vi "Append Text Table to Report.vi"(0 "report in":refnum<class "NI_Excel.lvclass">, 1 "column width (1)":dbl=1.0 format="%.2f", 2 "measurement system":u16(ring)=2 caption="measurement system for column width (Default)" items=["US", "Metric", "Default"], 3 "MS Office parameters":T2, 5 "column headers":string[](array[string]), 7 "row headers":string[](array[string]), 9 "text data":string[][](array[string]), 11 "error in (no error)":errorcluster, 13 "separate page?":bool, 14 "show grid lines":bool=TRUE) -> (4 "report out":refnum<class "NI_Excel.lvclass">, 8 "range (wd) - start (xl)":T1, 10 "end (xl)":cluster{"row (xl) ":i32, "col (xl) ":i32}, 15 "error out":errorcluster)   [LabVIEW 2023, in "NI_Excel.lvclass"]
doc: "Appends a 2D array to a report as a table with the given column width. You can use this polymorphic VI to append an array of strings or numbers. The data type you wire to the <B>text data</B> input determines the polymorphic instance to use."
uses:
  NI_Excel.lvclass
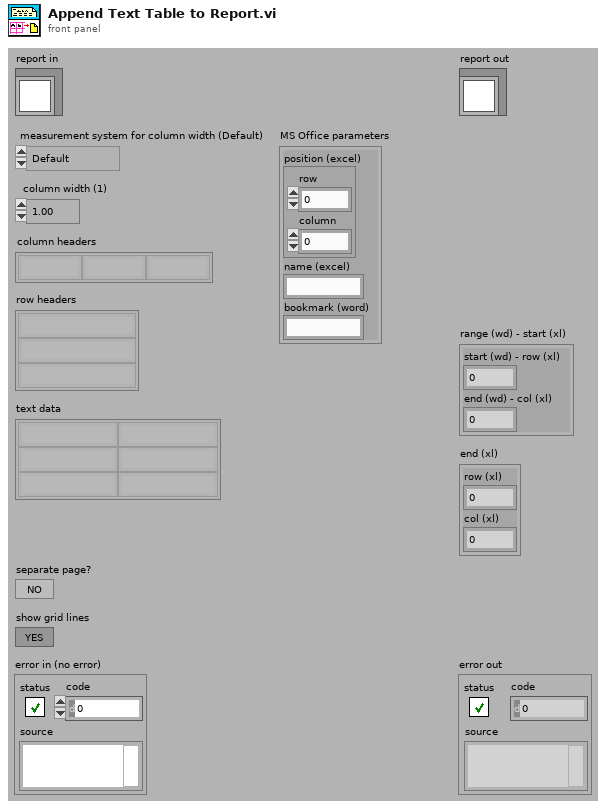
[diagram p1: front panel]
types:
  T1 = cluster{"start (wd) - row (xl) ":i32, "end (wd) - col (xl) ":i32}
  T2 = cluster{"position (excel)":cluster{"row":i32, "column":i32}, "name (excel)":string, "bookmark (word)":string}
  T3 = typedef "NI_ReportGenerationCore.lvlib/Report Data Members.ctl" = cluster{"font":T4, "from template?":bool}
  T4 = typedef "NI_ReportGenerationCore.lvlib/font.ctl" = cluster{"font name":string, "font size":dbl, "bold":u16, "italic":u16, "underline":u16, "strike through":u16, "font color":u32}
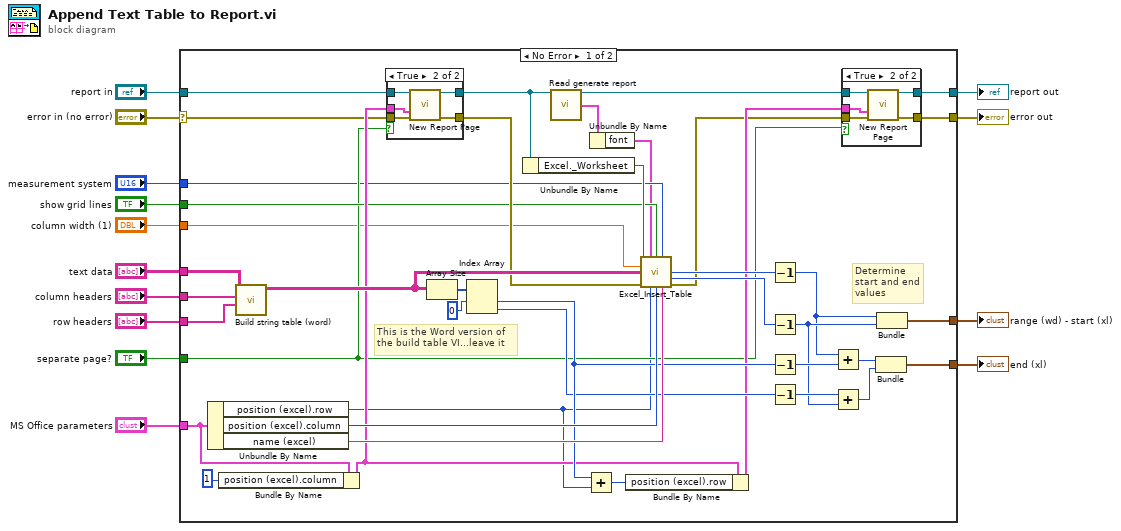
[diagram p0: block diagram]
diagram:
  n1 = case shown="No Error" "error in (no error)" {
    selector: "error in (no error)" -> [w34 w71]
    tunnel: [w33 w71] -> w13
    tunnel: [w30 w70] -> w11
    tunnel: "report in" -> [w35 w70]
    tunnel: "MS Office parameters" -> [w29 _]
    tunnel: [w28 _] -> w9
    tunnel: [w27 _] -> w8
    tunnel: "show grid lines" -> [w26 _]
    tunnel: "separate page?" -> [w25 _]
    tunnel: "text data" -> [w23 _]
    tunnel: "measurement system" -> [w22 _]
    tunnel: "column width (1)" -> [w21 _]
    tunnel: "column headers" -> [w20 _]
    tunnel: "row headers" -> [w19 _]
    frame No Error {
      # "This is the Word version of\nthe build table VI...leave it"
      # "Determine start and end values"
      n2 = Unbundle By Name(w29) -> ("position (excel).row"=w24:i32, "position (excel).column"=w54:i32, "name (excel)"=w55:string)
      n3 = Bundle By Name(cluster=w29, "position (excel).column"=1) -> (w36:T2)
      n4 = call <vilib>:"Build string table (word).vi"("row headers"=w19, "column headers"=w20, "text data"=w23) -> ("output table"=w50:string[][])  [unwired: 1 in, 7 out]
      n5 = case shown="True" w25 {
        tunnel: w35 -> [w64 w69]
        tunnel: w34 -> [w63 w68]
        tunnel: [w64 w67] -> w18
        tunnel: [w63 w66] -> w32
        tunnel: w36 -> [_ w65]
        frame False {
        }
        frame True {
          n6 = call-dynamic "New Report Page.vi"("report in"=w69, "MS Office parameters"=w65, "error in (no error)"=w68) -> ("report out"=w67:refnum<class "NI_Excel.lvclass">, "error out"=w66:errorcluster)  [unwired: 11 in]
        }
      }
      n7 = Array Size(array=w50) -> (size(s)=w40:i32[])
      n8 = Index Array(array=w40, index #1=0 ("Index")) -> (element #1=w53:i32, element #2=w48:i32)  [unwired: 1 in]
      n9 = Unbundle By Name(w18) -> ("Excel._Worksheet"=w49:refnum<k7>)
      n10 = call-dynamic "Read generate report.vi"("report in"=w18) -> ("report out"=w17:refnum<class "NI_Excel.lvclass">, "generate report"=w16:T3)  [unwired: 12 in, 1 out]
      n11 = Add(x=w53, y=w24) -> (x+y=w38:i32)
      n12 = Unbundle By Name(w16) -> ("font"=w15:T4)
      n13 = Bundle By Name(cluster=w36, "position (excel).row"=w38) -> (w39:T2)
      n14 = call <vilib>:"Excel_Insert_Table.vi"("worksheet"=w49, "font"=w15, "show grid lines"=w26, "measurement system"=w22, "column width (1)"=w21, "table"=w50, "error in (no error)"=w32, "Start row"=w24, "Start column"=w54, "name"=w55) -> ("Row"=w51:i32, "Column"=w52:i32, "error out"=w31:errorcluster)  [unwired: 3 out]
      n15 = Decrement(x=w51) -> (x-1=w44:i32)
      n16 = Decrement(x=w52) -> (x-1=w45:i32)
      n17 = Decrement(x=w53) -> (x-1=w46:i32)
      n18 = Decrement(x=w48) -> (x-1=w47:i32)
      n19 = Add(x=w44, y=w46) -> (x+y=w42:i32)
      n20 = Add(x=w47, y=w45) -> (x+y=w43:i32)
      n21 = case shown="True" w25 {
        tunnel: [w57 w62] -> w30
        tunnel: [w56 w61] -> w33
        tunnel: w31 -> [w56 w60]
        tunnel: w17 -> [w57 w59]
        tunnel: w39 -> [_ w58]
        frame False {
        }
        frame True {
          n22 = call-dynamic "New Report Page.vi"("report in"=w59, "MS Office parameters"=w58, "error in (no error)"=w60) -> ("report out"=w62:refnum<class "NI_Excel.lvclass">, "error out"=w61:errorcluster)  [unwired: 11 in]
        }
      }
      n23 = Bundle(w42, w43) -> (w27:cluster{i32, i32})  [unwired: 1 out]
      n24 = Bundle(w44, w45) -> (w28:cluster{i32, i32})  [unwired: 1 out]
    }
    frame Error {
    }
  }
  "error out" <- w13
  "report out" <- w11
  "end (xl)" <- w8
  "range (wd) - start (xl)" <- w9
